vi "iHR550 Read Values v10.6.2.vi"(1 "Mono Calibration":path, 2 "error in":errorcluster, 3 "JYMONOLib.IJYMonoReqd":refnum<k7>) -> (0 "iHR Current Values":T1={"iHR 550 Front Entrance"=0.0, "iHR550 Side Exit"=0.0, "iHR550 Wavelength"=897.9988, "iHR550 Exit Mirror"=2, "iHR550 Grating"="1", "Grating Index"=1} {"iHR550 Exit Mirror" items=["EntranceMirror", "ExitMirror", "Front", "Side"]})   [LabVIEW 2010]
uses:
  TypeDefs/iHR Current Values.ctl
panel:
  out "Current Description":string="1" caption="Description"
  out "Grating Index":i32=1
  out "Current Grating":dbl=1200.0
  out "error out":errorcluster
  out "Units 5":string="mm"
  out "Units 4":string="mm"
  out "Units 3":string="mm"
  out "Units 2":string="mm"
  out "Side Exit":dbl
  out "Front Exit":dbl
  out "Side Entrance":dbl
  out "Front Entrance":dbl
  out "Exit Mirror\nPosition":i32(ring)=2 items=["EntranceMirror", "ExitMirror", "Front", "Side"]
  out "Entrance Mirror\nPosition":i32(ring)=2 items=["EntranceMirror", "ExitMirror", "Front", "Side"]
  out "Units":string="nm"
  out "Current WL":dbl=897.9988
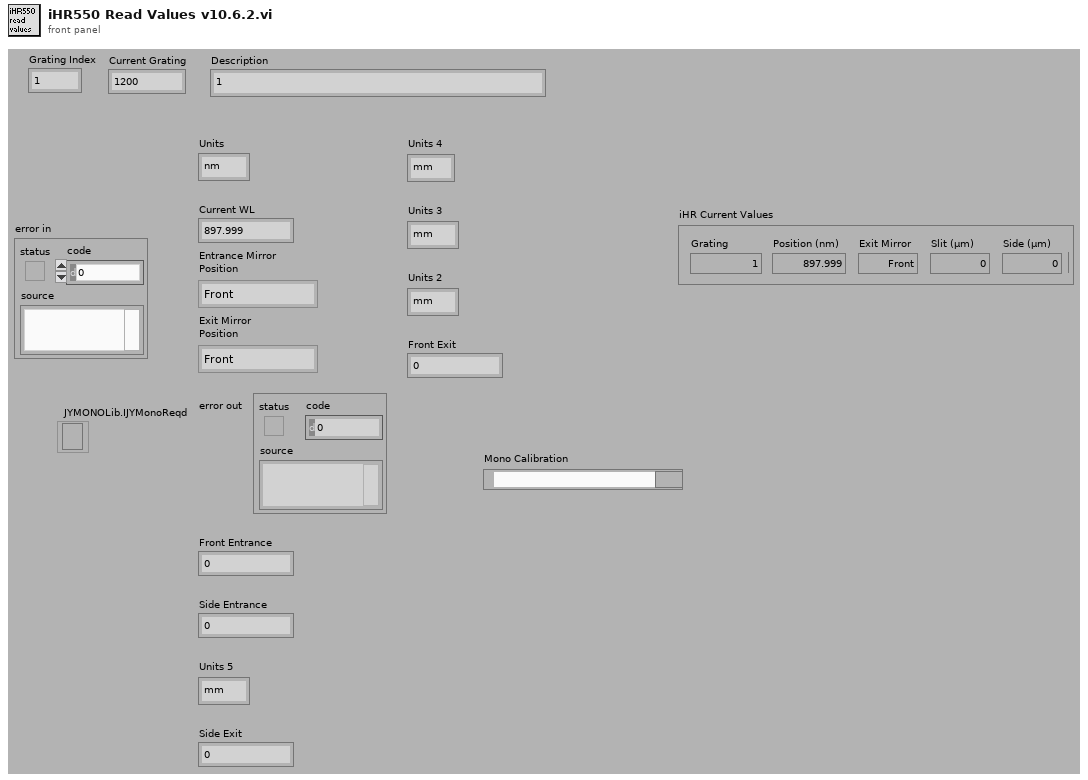
[diagram p1: front panel]
types:
  T1 = typedef "iHR Current Values.ctl" = cluster{"iHR 550 Front Entrance":dbl, "iHR550 Side Exit":dbl, "iHR550 Wavelength":dbl, "iHR550 Exit Mirror":i32, "iHR550 Grating":string, "Grating Index":i32}
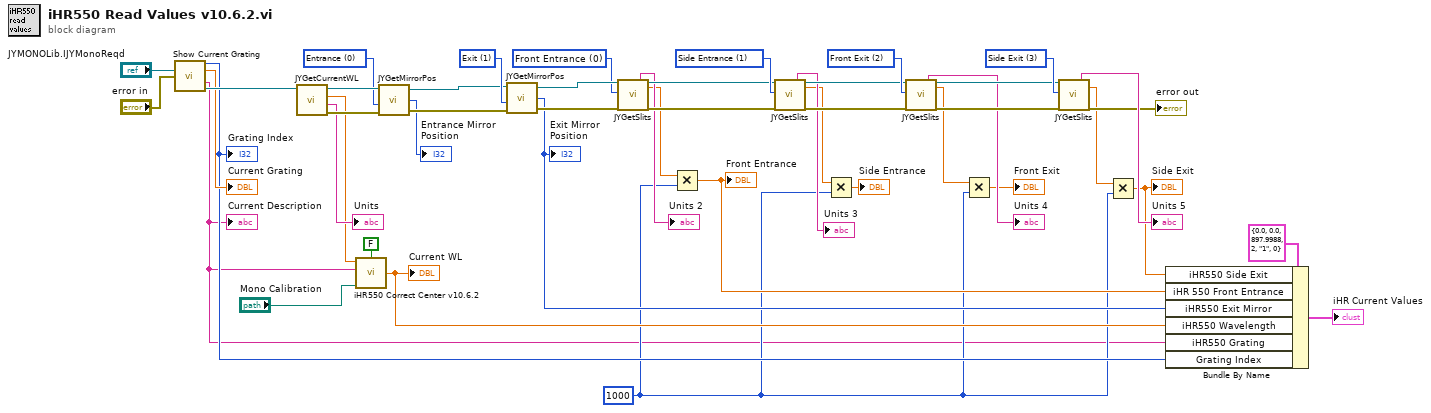
[diagram p0: block diagram]
diagram:
  w7 = i16 1000 ("y")
  w42 = u16 3 items=["Front Entrance", "Side Entrance", "Front Exit", "Side Exit", "First Intermediate", "Second Intermediate"] ("Slit")
  w43 = u16 2 items=["Front Entrance", "Side Entrance", "Front Exit", "Side Exit", "First Intermediate", "Second Intermediate"] ("Slit")
  w44 = u16 1 items=["Front Entrance", "Side Entrance", "Front Exit", "Side Exit", "First Intermediate", "Second Intermediate"] ("Slit")
  w45 = u16 0 items=["Front Entrance", "Side Entrance", "Front Exit", "Side Exit", "First Intermediate", "Second Intermediate"] ("Slit")
  w27 = u16 1 items=["Entrance", "Exit"] ("Mirror Number")
  w28 = u16 0 items=["Entrance", "Exit"] ("Mirror Number")
  n1 = call "Show Current Grating.vi"("Refnum in"="JYMONOLib.IJYMonoReqd", "error in (no error)"="error in") -> ("Grating Index"=w12:i32, "Current Grating"=→"Current Grating":dbl, "Current Description"=w2:string, "JYMONOLib.IJYMonoReqd"=w20:refnum<k7>)  [unwired: 5 in, 5 out]
  "Grating Index" <- w12
  "Current Description" <- w2
  n2 = call "JYGetCurrentWL.vi"("JYMONOLib.IJYMonoReqd"=w20) -> ("error out"=w30:errorcluster, "Units"=→"Units":string, "Current WL"=w13:dbl, "JYMONOLib.IJYMonoReqd 2"=w29:refnum<k7>)  [unwired: 7 in]
  n3 = call "iHR550 Correct Center v10.6.2.vi"("Calibration File"="Mono Calibration", "Set?"=FALSE, "Description"=w2, "Position In (nm)"=w13) -> ("Position Out (nm)"=w14:dbl)
  "Current WL" <- w14
  n4 = call "JYGetMirrorPos.vi"("error in (no error)"=w30, "Mirror"=w28, "Refnum In"=w29) -> ("error out"=w25:errorcluster, "Current Mirror Position"=→"Entrance Mirror\nPosition":i32, "Refnum Out"=w26:refnum<k7>)  [unwired: 1 in]
  n5 = call "JYGetMirrorPos.vi"("error in (no error)"=w25, "Mirror"=w27, "Refnum In"=w26) -> ("error out"=w46:errorcluster, "Current Mirror Position"=w17:i32, "Refnum Out"=w47:refnum<k7>)  [unwired: 1 in]
  "Exit Mirror\nPosition" <- w17
  n6 = call "JYGetSlits.vi"("MonoRefNum IN"=w47, "Slit"=w45, "error in (no error)"=w46) -> ("Units"=→"Units 2":string, "MonoRefNum Out"=w41:refnum<k7>, "Slit Width"=w11:dbl, "error out"=w38:errorcluster)  [unwired: 13 in]
  n7 = Multiply(x=w11, y=w7) -> (x*y=w8:dbl)
  "Front Entrance" <- w8
  n8 = call "JYGetSlits.vi"("MonoRefNum IN"=w41, "Slit"=w44, "error in (no error)"=w38) -> ("Units"=→"Units 3":string, "MonoRefNum Out"=w40:refnum<k7>, "Slit Width"=w10:dbl, "error out"=w37:errorcluster)  [unwired: 13 in]
  n9 = Multiply(x=w10, y=w7) -> (x*y=→"Side Entrance":dbl)
  n10 = call "JYGetSlits.vi"("MonoRefNum IN"=w40, "Slit"=w43, "error in (no error)"=w37) -> ("Units"=→"Units 4":string, "MonoRefNum Out"=w39:refnum<k7>, "Slit Width"=w3:dbl, "error out"=w36:errorcluster)  [unwired: 13 in]
  n11 = Multiply(x=w3, y=w7) -> (x*y=→"Front Exit":dbl)
  n12 = call "JYGetSlits.vi"("MonoRefNum IN"=w39, "Slit"=w42, "error in (no error)"=w36) -> ("Units"=→"Units 5":string, "Slit Width"=w4:dbl, "error out"=→"error out":errorcluster)  [unwired: 13 in, 1 out]
  n13 = Multiply(x=w4, y=w7) -> (x*y=w5:dbl)
  "Side Exit" <- w5
  n14 = Bundle By Name(cluster=T1 {"iHR 550 Front Entrance"=0.0, "iHR550 Side Exit"=0.0, "iHR550 Wavelength"=897.9988, "iHR550 Exit Mirror"=2, "iHR550 Grating"="1", "Grating Index"=0} ("iHR Current Values"), "iHR550 Side Exit"=w5, "iHR 550 Front Entrance"=w8, "iHR550 Exit Mirror"=w17, "iHR550 Wavelength"=w14, "iHR550 Grating"=w2, "Grating Index"=w12) -> (→"iHR Current Values":T1)
